vi "Trion Simulation.vi"(2 "Array":cluster{"Vsg":dbl[], "B":dbl[]}[](array[cluster])=[{"Vsg"=[0.14, 0.31, 0.42, 0.55], "B"=[4.0, 6.0, 8.0, 9.0]}, {"Vsg"=[0.22, 0.31, 0.42, 0.48], "B"=[4.0, 6.0, 8.0, 9.0]}, {"Vsg"=[0.28, 0.31, 0.42, 0.43], "B"=[4.0, 6.0, 8.0, 9.0]}], 3 "frac":dbl) -> (0 "Intensity Graph":dbl[][](graph), 1 "XY Graph":cluster{"B":dbl[], "Vsg":dbl[]}[](graph)=[{"B"=[4.0, 4.1, 4.2, 4.3, 4.4, 4.5, 4.6, 4.7, 4.8, 4.9, 5.0, 5.1, 5.2, 5.3, 5.4, 5.5, 5.6, 5.7, 5.8, 5.9, 6.0, 6.1, 6.2, 6.300000000000001, 6.4, 6.5, 6.6, 6.7, 6.800000000000001, 6.9, 7.0, 7.1, 7.2, 7.300000000000001, 7.4, 7.5, 7.6, 7.7, 7.800000000000001, 7.9, 8.0, 8.100000000000001, 8.2, 8.3, 8.4, 8.5, 8.600000000000001, 8.7, 8.8, 8.9], "Vsg"=[0.14, 0.1485, 0.15700000000000003, 0.16549999999999998, 0.17400000000000004, 0.1825, 0.19099999999999998, 0.1995, 0.208, 0.21650000000000003, 0.225, 0.23349999999999999, 0.24200000000000002, 0.2505, 0.259, 0.2675, 0.27599999999999997, 0.2845, 0.293, 0.3015, 0.31, 0.3155, 0.321, 0.3265, 0.332, 0.3375, 0.34299999999999997, 0.34850000000000003, 0.35400000000000004, 0.35950000000000004, 0.365, 0.37049999999999994, 0.376, 0.38150000000000006, 0.387, 0.39249999999999996, 0.39799999999999996, 0.40349999999999997, 0.40900000000000003, 0.4145, 0.42, 0.43300000000000016, 0.4459999999999999, 0.4590000000000001, 0.47200000000000003, 0.485, 0.4980000000000002, 0.5109999999999999, 0.5240000000000001, 0.5370000000000001]}, {"B"=[4.0, 4.1, 4.2, 4.3, 4.4, 4.5, 4.6, 4.7, 4.8, 4.9, 5.0, 5.1, 5.2, 5.3, 5.4, 5.5, 5.6, 5.7, 5.8, 5.9, 6.0, 6.1, 6.2, 6.300000000000001, 6.4, 6.5, 6.6, 6.7, 6.800000000000001, 6.9, 7.0, 7.1, 7.2, 7.300000000000001, 7.4, 7.5, 7.6, 7.7, 7.800000000000001, 7.9, 8.0, 8.100000000000001, 8.2, 8.3, 8.4, 8.5, 8.600000000000001, 8.7, 8.8, 8.9], "Vsg"=[0.22, 0.22449999999999998, 0.229, 0.23349999999999999, 0.23800000000000002, 0.2425, 0.247, 0.2515, 0.256, 0.2605, 0.265, 0.26949999999999996, 0.274, 0.27849999999999997, 0.28300000000000003, 0.2875, 0.292, 0.2965, 0.301, 0.3055, 0.31, 0.3155, 0.321, 0.3265, 0.332, 0.3375, 0.34299999999999997, 0.34850000000000003, 0.35400000000000004, 0.35950000000000004, 0.365, 0.37049999999999994, 0.376, 0.38150000000000006, 0.387, 0.39249999999999996, 0.39799999999999996, 0.40349999999999997, 0.40900000000000003, 0.4145, 0.42, 0.42600000000000005, 0.43199999999999994, 0.438, 0.444, 0.44999999999999996, 0.45600000000000007, 0.46199999999999997, 0.468, 0.474]}, {"B"=[4.0, 4.1, 4.2, 4.3, 4.4, 4.5, 4.6, 4.7, 4.8, 4.9, 5.0, 5.1, 5.2, 5.3, 5.4, 5.5, 5.6, 5.7, 5.8, 5.9, 6.0, 6.1, 6.2, 6.300000000000001, 6.4, 6.5, 6.6, 6.7, 6.800000000000001, 6.9, 7.0, 7.1, 7.2, 7.300000000000001, 7.4, 7.5, 7.6, 7.7, 7.800000000000001, 7.9, 8.0, 8.100000000000001, 8.2, 8.3, 8.4, 8.5, 8.600000000000001, 8.7, 8.8, 8.9], "Vsg"=[0.28, 0.28150000000000003, 0.28300000000000003, 0.28450000000000003, 0.28600000000000003, 0.28750000000000003, 0.28900000000000003, 0.29050000000000004, 0.29200000000000004, 0.29350000000000004, 0.29500000000000004, 0.2965, 0.298, 0.2995, 0.301, 0.3025, 0.304, 0.3055, 0.307, 0.3085, 0.31, 0.3155, 0.321, 0.3265, 0.332, 0.3375, 0.34299999999999997, 0.34850000000000003, 0.35400000000000004, 0.35950000000000004, 0.365, 0.37049999999999994, 0.376, 0.38150000000000006, 0.387, 0.39249999999999996, 0.39799999999999996, 0.40349999999999997, 0.40900000000000003, 0.4145, 0.42, 0.421, 0.422, 0.423, 0.424, 0.425, 0.426, 0.427, 0.428, 0.429]}])   [LabVIEW 2016]
panel:
  in  "dV":dbl=0.001
  in  "NV":dbl=900.0
  in  "V0":dbl
  in  "width":dbl=0.03
  in  "noise":dbl=0.05
  out "B":dbl[](array[numeric])=[4.0, 6.0, 8.0, 9.0]
  out "Vsg":dbl[](array[numeric])=[0.28, 0.31, 0.42, 0.43]
  out "Interpolated":cluster{"Vsg":dbl[], "B":dbl[]}[](array[cluster])=[{"Vsg"=[0.14, 0.22, 0.28], "B"=[4.0, 4.0, 4.0]}, {"Vsg"=[0.1485, 0.22449999999999998, 0.28150000000000003], "B"=[4.1, 4.1, 4.1]}, {"Vsg"=[0.15700000000000003, 0.229, 0.28300000000000003], "B"=[4.2, 4.2, 4.2]}, {"Vsg"=[0.16549999999999998, 0.23349999999999999, 0.28450000000000003], "B"=[4.3, 4.3, 4.3]}, {"Vsg"=[0.17400000000000004, 0.23800000000000002, 0.28600000000000003], "B"=[4.4, 4.4, 4.4]}, {"Vsg"=[0.1825, 0.2425, 0.28750000000000003], "B"=[4.5, 4.5, 4.5]}, {"Vsg"=[0.19099999999999998, 0.247, 0.28900000000000003], "B"=[4.6, 4.6, 4.6]}, {"Vsg"=[0.1995, 0.2515, 0.29050000000000004], "B"=[4.7, 4.7, 4.7]}, {"Vsg"=[0.208, 0.256, 0.29200000000000004], "B"=[4.8, 4.8, 4.8]}, {"Vsg"=[0.21650000000000003, 0.2605, 0.29350000000000004], "B"=[4.9, 4.9, 4.9]}, {"Vsg"=[0.225, 0.265, 0.29500000000000004], "B"=[5.0, 5.0, 5.0]}, {"Vsg"=[0.23349999999999999, 0.26949999999999996, 0.2965], "B"=[5.1, 5.1, 5.1]}, {"Vsg"=[0.24200000000000002, 0.274, 0.298], "B"=[5.2, 5.2, 5.2]}, {"Vsg"=[0.2505, 0.27849999999999997, 0.2995], "B"=[5.3, 5.3, 5.3]}, {"Vsg"=[0.259, 0.28300000000000003, 0.301], "B"=[5.4, 5.4, 5.4]}, {"Vsg"=[0.2675, 0.2875, 0.3025], "B"=[5.5, 5.5, 5.5]}, {"Vsg"=[0.27599999999999997, 0.292, 0.304], "B"=[5.6, 5.6, 5.6]}, {"Vsg"=[0.2845, 0.2965, 0.3055], "B"=[5.7, 5.7, 5.7]}, {"Vsg"=[0.293, 0.301, 0.307], "B"=[5.8, 5.8, 5.8]}, {"Vsg"=[0.3015, 0.3055, 0.3085], "B"=[5.9, 5.9, 5.9]}, {"Vsg"=[0.31, 0.31, 0.31], "B"=[6.0, 6.0, 6.0]}, {"Vsg"=[0.3155, 0.3155, 0.3155], "B"=[6.1, 6.1, 6.1]}, {"Vsg"=[0.321, 0.321, 0.321], "B"=[6.2, 6.2, 6.2]}, {"Vsg"=[0.3265, 0.3265, 0.3265], "B"=[6.300000000000001, 6.300000000000001, 6.300000000000001]}, {"Vsg"=[0.332, 0.332, 0.332], "B"=[6.4, 6.4, 6.4]}, {"Vsg"=[0.3375, 0.3375, 0.3375], "B"=[6.5, 6.5, 6.5]}, {"Vsg"=[0.34299999999999997, 0.34299999999999997, 0.34299999999999997], "B"=[6.6, 6.6, 6.6]}, {"Vsg"=[0.34850000000000003, 0.34850000000000003, 0.34850000000000003], "B"=[6.7, 6.7, 6.7]}, {"Vsg"=[0.35400000000000004, 0.35400000000000004, 0.35400000000000004], "B"=[6.800000000000001, 6.800000000000001, 6.800000000000001]}, {"Vsg"=[0.35950000000000004, 0.35950000000000004, 0.35950000000000004], "B"=[6.9, 6.9, 6.9]}, {"Vsg"=[0.365, 0.365, 0.365], "B"=[7.0, 7.0, 7.0]}, {"Vsg"=[0.37049999999999994, 0.37049999999999994, 0.37049999999999994], "B"=[7.1, 7.1, 7.1]}, {"Vsg"=[0.376, 0.376, 0.376], "B"=[7.2, 7.2, 7.2]}, {"Vsg"=[0.38150000000000006, 0.38150000000000006, 0.38150000000000006], "B"=[7.300000000000001, 7.300000000000001, 7.300000000000001]}, {"Vsg"=[0.387, 0.387, 0.387], "B"=[7.4, 7.4, 7.4]}, {"Vsg"=[0.39249999999999996, 0.39249999999999996, 0.39249999999999996], "B"=[7.5, 7.5, 7.5]}, {"Vsg"=[0.39799999999999996, 0.39799999999999996, 0.39799999999999996], "B"=[7.6, 7.6, 7.6]}, {"Vsg"=[0.40349999999999997, 0.40349999999999997, 0.40349999999999997], "B"=[7.7, 7.7, 7.7]}, {"Vsg"=[0.40900000000000003, 0.40900000000000003, 0.40900000000000003], "B"=[7.800000000000001, 7.800000000000001, 7.800000000000001]}, {"Vsg"=[0.4145, 0.4145, 0.4145], "B"=[7.9, 7.9, 7.9]}, {"Vsg"=[0.42, 0.42, 0.42], "B"=[8.0, 8.0, 8.0]}, {"Vsg"=[0.43300000000000016, 0.42600000000000005, 0.421], "B"=[8.100000000000001, 8.100000000000001, 8.100000000000001]}, {"Vsg"=[0.4459999999999999, 0.43199999999999994, 0.422], "B"=[8.2, 8.2, 8.2]}, {"Vsg"=[0.4590000000000001, 0.438, 0.423], "B"=[8.3, 8.3, 8.3]}, {"Vsg"=[0.47200000000000003, 0.444, 0.424], "B"=[8.4, 8.4, 8.4]}, {"Vsg"=[0.485, 0.44999999999999996, 0.425], "B"=[8.5, 8.5, 8.5]}, {"Vsg"=[0.4980000000000002, 0.45600000000000007, 0.426], "B"=[8.600000000000001, 8.600000000000001, 8.600000000000001]}, {"Vsg"=[0.5109999999999999, 0.46199999999999997, 0.427], "B"=[8.7, 8.7, 8.7]}, {"Vsg"=[0.5240000000000001, 0.468, 0.428], "B"=[8.8, 8.8, 8.8]}, {"Vsg"=[0.5370000000000001, 0.474, 0.429], "B"=[8.9, 8.9, 8.9]}]
  in  "NB":dbl=50.0
  in  "dB":dbl=0.1
  in  "B0":dbl=4.0
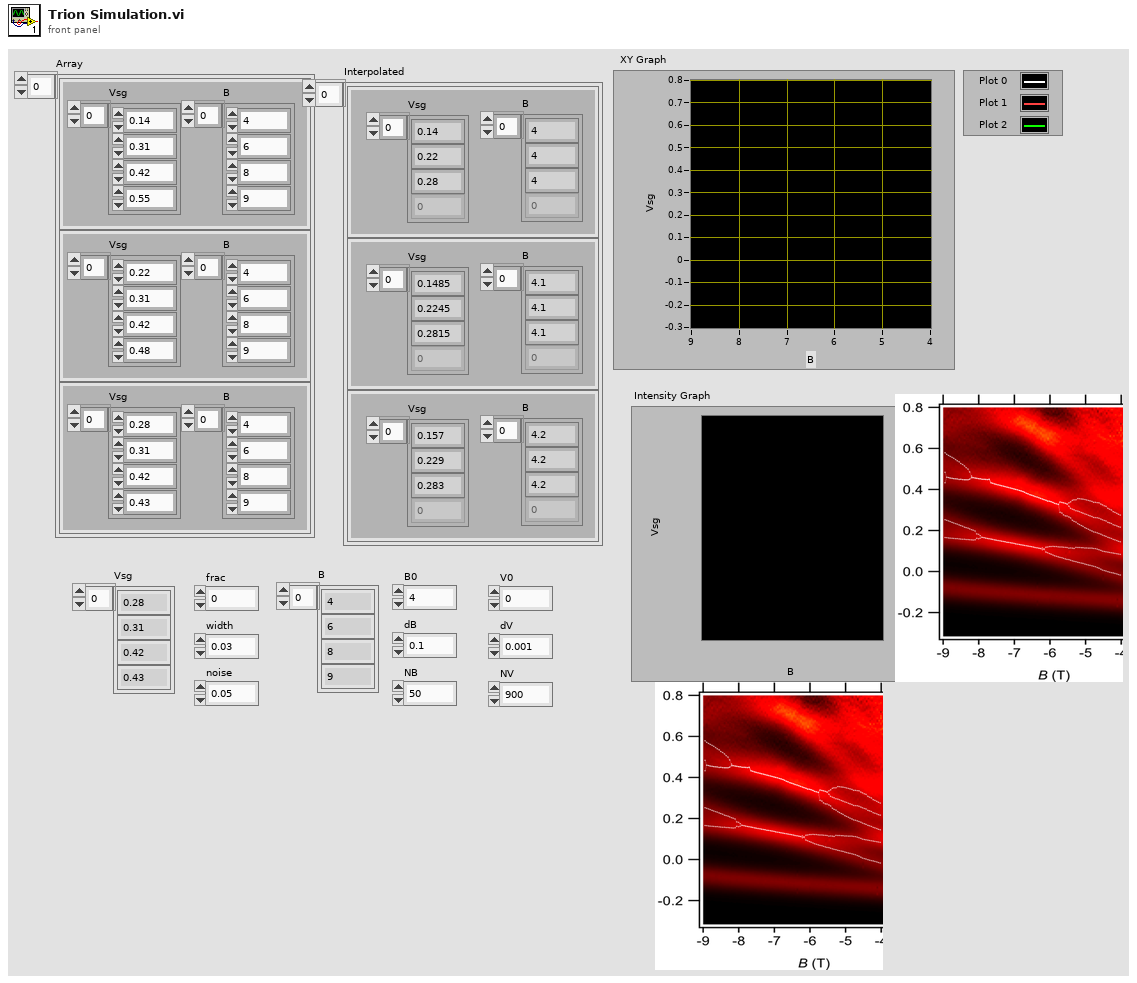
[diagram p1: front panel]
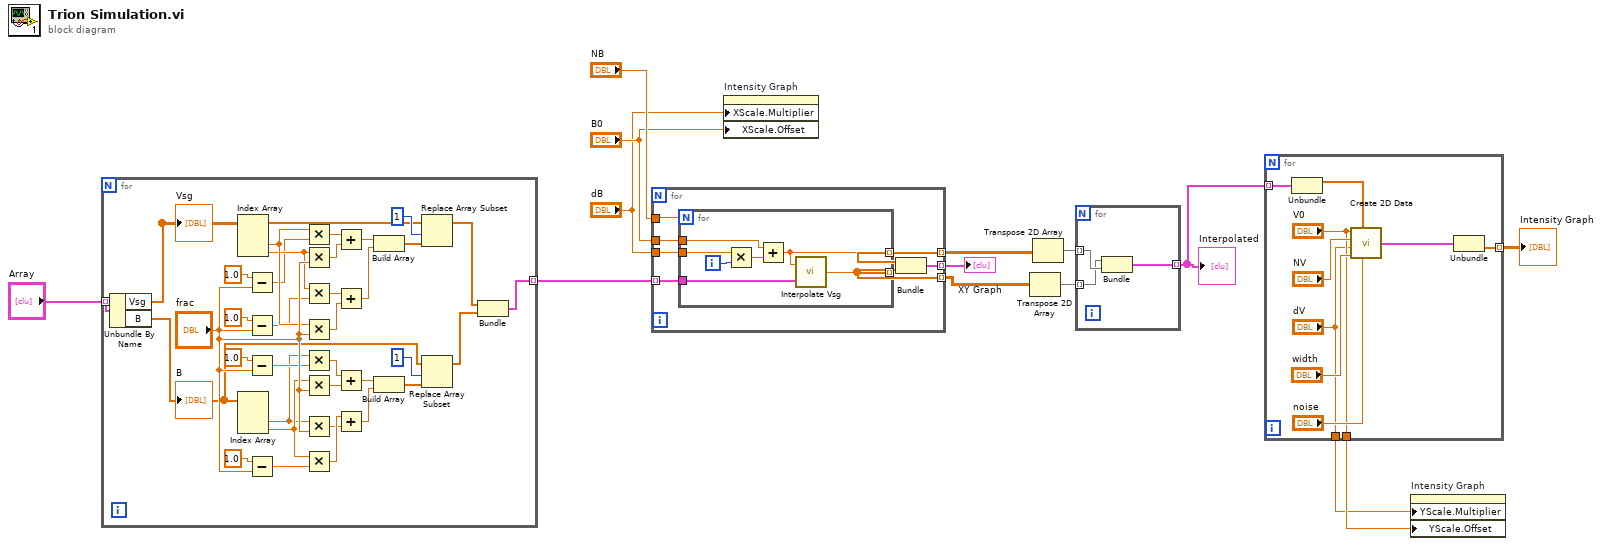
[diagram p0: block diagram]
diagram:
  n1 = for {
    tunnel: "Array" -> [w20] mode=indexing
    tunnel: [w16] -> w5 mode=indexing
    n2 = Unbundle By Name(w20) -> ("Vsg"=w15:dbl[], "B"=w19:dbl[])
    "Vsg" <- w15
    "B" <- w19
    n3 = Index Array(array=w15) -> (element #2=w30:dbl, element #3=w29:dbl)  [unwired: 3 in, 1 out]
    n4 = Index Array(array=w19) -> (element #2=w39:dbl, element #3=w40:dbl)  [unwired: 3 in, 1 out]
    n5 = Subtract(x=1.0, y="frac") -> (x-y=w22:dbl)
    n6 = Subtract(x=1.0, y="frac") -> (x-y=w27:dbl)
    n7 = Subtract(x=1.0, y="frac") -> (x-y=w47:dbl)
    n8 = Subtract(x=1.0, y="frac") -> (x-y=w42:dbl)
    n9 = Multiply(x=w30, y=w22) -> (x*y=w24:dbl)
    n10 = Multiply(x=w29, y="frac") -> (x*y=w23:dbl)
    n11 = Multiply(x=w29, y=w27) -> (x*y=w25:dbl)
    n12 = Multiply(x=w30, y="frac") -> (x*y=w26:dbl)
    n13 = Multiply(x=w39, y=w47) -> (x*y=w45:dbl)
    n14 = Multiply(x=w40, y="frac") -> (x*y=w46:dbl)
    n15 = Multiply(x=w39, y="frac") -> (x*y=w43:dbl)
    n16 = Multiply(x=w40, y=w42) -> (x*y=w44:dbl)
    n17 = Add(x=w24, y=w23) -> (x+y=w32:dbl)
    n18 = Add(x=w25, y=w26) -> (x+y=w31:dbl)
    n19 = Add(x=w45, y=w46) -> (x+y=w37:dbl)
    n20 = Add(x=w44, y=w43) -> (x+y=w38:dbl)
    n21 = Build Array(w32, w31) -> (w34:dbl[])
    n22 = Build Array(w37, w38) -> (w35:dbl[])
    n23 = Replace Array Subset(array=w15, new element=w34, index=1) -> (w17:dbl[])
    n24 = Replace Array Subset(array=w19, new element=w35, index=1) -> (w18:dbl[])
    n25 = Bundle("Vsg"=w17, "B"=w18) -> (w16:cluster{"Vsg":dbl[], "B":dbl[]})  [unwired: 1 in]
  }
  n26 = for {
    tunnel: w5 -> [w56] mode=indexing
    tunnel: "dB" -> [w55]
    tunnel: "B0" -> [w54]
    tunnel: "NB" -> [w53]
    tunnel: [w52] -> w13 mode=indexing
    tunnel: [w51] -> w11 mode=indexing
    tunnel: [w50] -> w12 mode=indexing
    n27 = for {
      N: w53 -> [_]
      tunnel: w56 -> [w57]
      tunnel: w55 -> [w62]
      tunnel: w54 -> [w60]
      tunnel: [w59] -> w50 mode=indexing
      tunnel: [w58] -> w51 mode=indexing
      i -> [w63]
      n28 = Multiply(x=w62, y=w63) -> (x*y=w61:dbl)
      n29 = Add(x=w60, y=w61) -> (x+y=w58:dbl)
      n30 = call "Interpolate Vsg.vi"("Vsg(B)"=w57, "B"=w58) -> ("Vsg"=w59:dbl)
    }
    n31 = Bundle(w51, w50) -> (w52:cluster{dbl[], dbl[]})  [unwired: 1 in]
  }
  "XY Graph" <- w13
  n32 = property on="Intensity Graph" class="IntGraph (strict)"("XScale.Multiplier"="dB", "XScale.Offset"="B0") -> ()  [unwired: 2 in, 2 out]
  n33 = Transpose 2D Array(2D array=w12) -> (transposed array=w9:dbl[][])
  n34 = Transpose 2D Array(2D array=w11) -> (transposed array=w10:dbl[][])
  n35 = for {
    tunnel: w10 -> [w65] mode=indexing
    tunnel: w9 -> [w64] mode=indexing
    tunnel: [w66] -> w8 mode=indexing
    n36 = Bundle(w64, w65) -> (w66:cluster{dbl[], dbl[]})  [unwired: 1 in]
  }
  "Interpolated" <- w8
  n37 = for {
    tunnel: w8 -> [w75] mode=indexing
    tunnel: [w72] -> w7 mode=indexing
    tunnel: ["V0"] -> w2
    tunnel: ["dV"] -> w1
    n38 = Unbundle(w75) -> (w74:dbl[])  [unwired: 1 out]
    n39 = call "Create 2D Data.vi"("noise"="noise", "Vsg"=w74, "width"="width", "dV"="dV", "NV"="NV", "V0"="V0") -> ("XY Graph"=w73:cluster{dbl[], dbl[]})
    n40 = Unbundle(w73) -> (w72:dbl[])  [unwired: 1 out]
  }
  "Intensity Graph" <- w7
  n41 = property on="Intensity Graph" class="IntGraph (strict)"("YScale.Multiplier"=w1, "YScale.Offset"=w2) -> ()  [unwired: 2 in, 2 out]
